vi "addLayout.vi"(4 "columnSpan (1)":i32=1, 5 "rowSpan (1)":i32=1, 6 "column":i32, 7 "row":i32, 8 "Error In":errorcluster, 10 "widget":refnum<class "QLayout.lvclass">, 11 "QGridLayout In":refnum<class "QGridLayout.lvclass">) -> (0 "Error Out":errorcluster, 3 "QGridLayout Out":refnum<class "QGridLayout.lvclass">)   [LabVIEW 2014, in "QGridLayout.lvclass"]
doc: "LabVIEW-specific documentation is not yet available. See <b>http://doc.qt.io/qt-5/QGridLayout.html#addLayout</b>"
uses:
  QGridLayout.lvclass
  QLayout/QLayout.lvclass
  LQ Core/LQIdentity/LQIdentity.lvclass/LQIdentity.ctl
  LQ Core/LQ Core.lvlib
  LQ Core/LQIdentity/LQIdentity.lvclass
panel:
  # "Copyright (c) 2016 Sze Howe Koh\n\nThis Source Code Form is subject to the terms of the Mozilla Public\nLicense, v. 2.0. If a copy of the MPL was not distributed with this\nfile, You can obtain one at http://mozilla.org/MPL/2.0/."
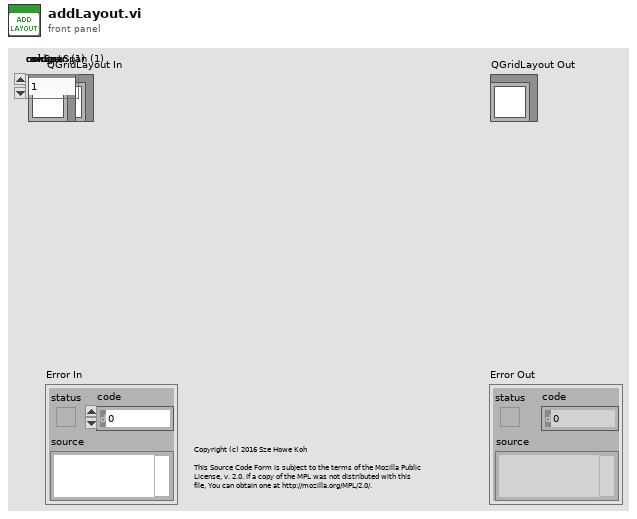
[diagram p1: front panel]
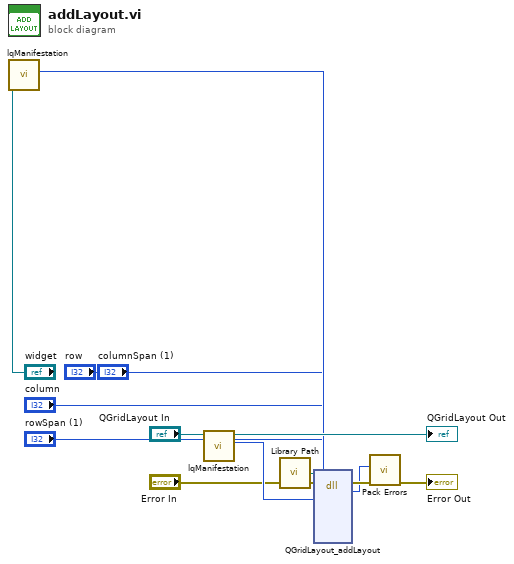
[diagram p0: block diagram]
diagram:
  n1 = call "lqManifestation.vi"("LQIdentity in"="widget") -> ("Manifestation"=w5:u64)  [unwired: 9 in, 1 out]
  n2 = call "lqManifestation.vi"("LQIdentity in"="QGridLayout In") -> ("Manifestation"=w11:u64, "LQIdentity out"=→"QGridLayout Out":refnum<class "QGridLayout.lvclass">)  [unwired: 9 in]
  n3 = call "Library Path.vi"() -> ("Library Path"=w12:path)
  n4 = dll-call lib="?" fn="QGridLayout_addLayout"(path in=w12, error in="Error In", "_instance"=w11, "widget"=w5, "row"="row", "column"="column", "rowSpan"="rowSpan (1)", "columnSpan"="columnSpan (1)") -> (error out=w9:errorcluster, w7:i32)  [unwired: 7 in, 1 out]
  n5 = call "Pack Errors.vi"("Error In"=w9, "Error Code"=w7) -> ("Error Out"=→"Error Out":errorcluster)  [unwired: 9 in]
